vi "Encoder Turn Short.vi"(10 "Setpoint":dbl=40.0 format="%.2f", 11 "Execute?":bool) -> (2 "output":dbl format="%.2f", 3 "Done":bool)   [LabVIEW 2012]
uses:
  <vilib>/addons/control/pid/pid.llb/PID (DBL).vi
  <vilib>/addons/control/pid/NI_PID_pid.lvlib
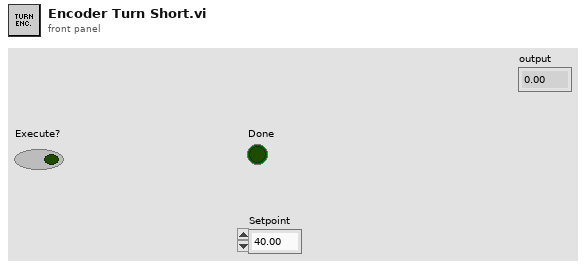
[diagram p1: front panel]
types:
  T1 = typedef "WPI_EncoderDevRef.ctl" = cluster{"DevStatus":errorcluster, "EncoderIndex":T2, "CounterIndex":T3, "DistancePerCount":dbl, "Decoding Type":T4}
  T2 = typedef "FPGA_EncoderIdx.ctl" = enum8{"Enc 0", "Enc 1", "Enc 2", "Enc 3", "Invalid"}
  T3 = typedef "FPGA_CounterCtrSystemIndex.ctl" = enum8{"Ctr 0", "Ctr 1", "Ctr 2", "Ctr 3", "Ctr 4", "Ctr 5", "Ctr 6", "Ctr 7", "Invalid"}
  T4 = typedef "WPI_EncoderType.ctl" = enum16{"1x", "2x", "4x"}
  T5 = cluster{"proportional gain (Kc)":dbl, "integral time (Ti, min)":dbl, "derivative time (Td, min)":dbl}
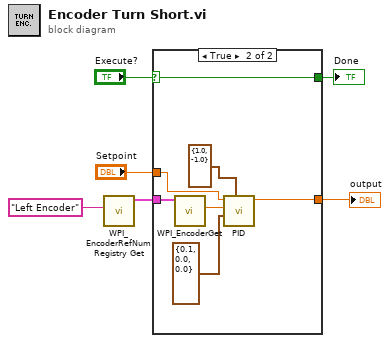
[diagram p0: block diagram]
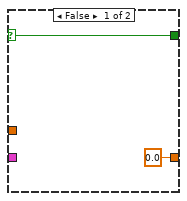
[diagram p2: hidden frame]
diagram:
  n1 = call <vilib>:"WPI_EncoderRefNum Registry Get.vi"("refnum name"="Left Encoder") -> ("EncoderDevRef"=w3:T1)  [unwired: 9 in, 1 out]
  n2 = case shown="True" "Execute?" {
    selector: "Execute?" -> [w8 w15]
    tunnel: [w8 w15] -> w4
    tunnel: w3 -> [_ w12]
    tunnel: "Setpoint" -> [_ w10]
    tunnel: [0.0 ("output") w9] -> w1
    frame False {
    }
    frame True {
      n3 = call <vilib>:"WPI_EncoderGet.vi"("EncoderDevRef"=w12) -> ("Distance"=w11:dbl)  [unwired: 5 in, 5 out]
      n4 = call-poly <vilib>:"PID.vi"("output range"=cluster{"output high":dbl, "output low":dbl} {"output high"=1.0, "output low"=-1.0}, "PID gains"=T5 {"proportional gain (Kc)"=0.1, "integral time (Ti, min)"=0.0, "derivative time (Td, min)"=0.0}, "process variable"=w11, "setpoint"=w10) -> ("output"=w9:dbl)  [unwired: 6 in, 1 out]
    }
  }
  "Done" <- w4
  "output" <- w1
